vi "controlVoltagesCalc.vi"(0 "Camera":T1 {"InClusTiming 2"."TriggerMode" items=["Auto", "Software", "External sequence start ", "External exposure control"]; "InClusTiming 2"."ExposureTimeBase" items=["nanoseconds", "microseconds", "milliseconds"]; "InClusTiming 2"."Pixelclock" min=1 max=150 step=1 scale=0.05915..150.0; "InClusTiming 2"."Framerate" min=0.05915 max=2000.0 step=1.0 scale=0.05915..100.0 scale format="%#.3g"; "InClusTiming 2"."Exposure" min=0.001 max=400.0 step=0.001 scale=0.05915..400.0 scale format="%#.3g"}, 7 "clustPointagFin":T2, 11 "error in (no error)":errorcluster) -> (4 "output cluster":T1={"Camera.lvclass"=refnum, "InClusTiming 2"={"Pixelclock"=24, "Exposure"=46.39115, "ExposureTimeBase"=2, "Framerate"=14.99615, "TriggerMode"=0}, "ROI"={"PosX"=0, "PosY"=0, "Width"=0, "Height"=0}, "File Path Control"=path "", "mirror.lvclass"=refnum} {"InClusTiming 2"."TriggerMode" items=["Auto", "Software", "External sequence start ", "External exposure control"]; "InClusTiming 2"."ExposureTimeBase" items=["nanoseconds", "microseconds", "milliseconds"]; "InClusTiming 2"."Pixelclock" min=1 max=150 step=1 scale=0.05915..150.0; "InClusTiming 2"."Framerate" min=0.05915 max=2000.0 step=1.0 scale=0.05915..100.0 scale format="%#.3g"; "InClusTiming 2"."Exposure" min=0.001 max=400.0 step=0.001 scale=0.05915..400.0 scale format="%#.3g"}, 8 "clustPointagFin":T2, 15 "error out":errorcluster)   [LabVIEW 2020, in "Acquisition.lvlib"]
doc: "Perform the acquisition. Replace the contents of this diagram with calls to acquisition hardware."
uses:
  Acquisition.lvlib
  CLASS/Image Acquisition Class/Camera.lvclass
  MIRROR/mirror.lvclass
  SETTING/clustOA.ctl
  <vilib>/Analysis/Matrix/Datatypes/RealMatrix.ctl
  HardwareConfiguration.ctl
  <vilib>/Analysis/Matrix/Numeric/Conversions/Array To Matrix - RA.vi
  <vilib>/Analysis/Matrix/Numeric/Multiply/Multiply - RM,RM.vi
  <vilib>/Analysis/Matrix/Numeric/Conversions/Matrix To Array - RM.vi
  <vilib>/Analysis/Matrix/NI_Matrix.lvlib
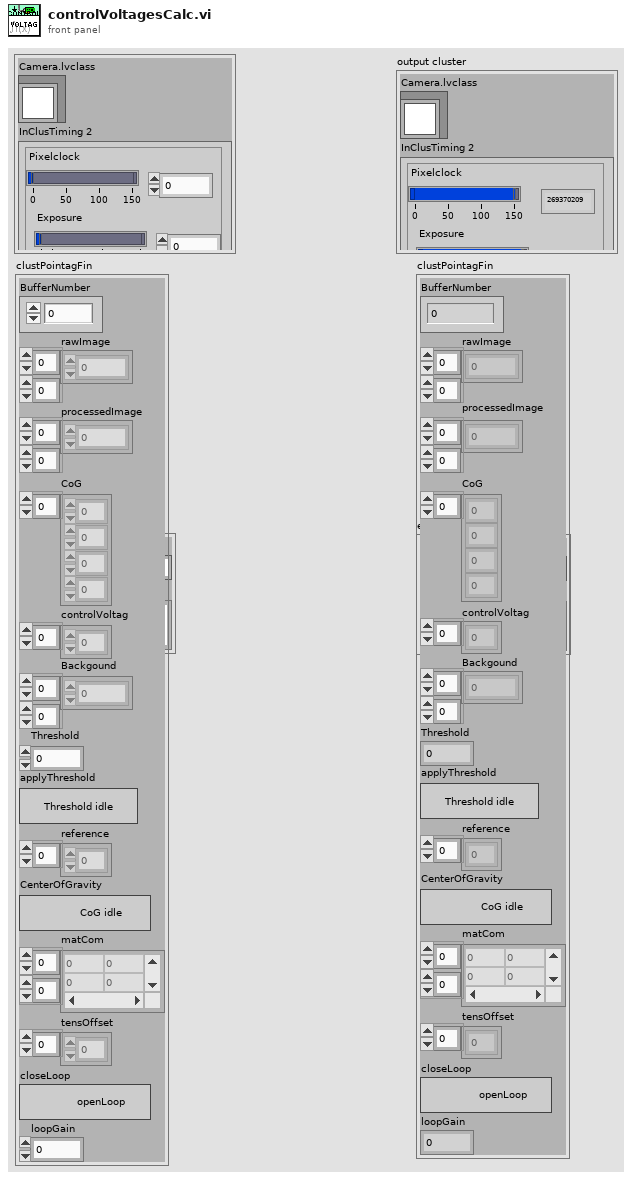
[diagram p1: front panel]
types:
  T1 = typedef "Acquisition.lvlib/HardwareConfiguration.ctl" = cluster{"Camera.lvclass":refnum<class "Camera.lvclass">, "InClusTiming 2":cluster{"Pixelclock":i32, "Exposure":dbl, "ExposureTimeBase":u16, "Framerate":dbl, "TriggerMode":u16}, "ROI":cluster{"PosX":i32, "PosY":i32, "Width":i32, "Height":i32}, "File Path Control":path, "mirror.lvclass":refnum<class "mirror.lvclass">}
  T2 = typedef "clustOA.ctl" = cluster{"BufferNumber":u32, "rawImage":u16[][], "processedImage":sgl[][], "CoG":dbl[], "controlVoltag":dbl[], "Backgound":sgl[][], "Threshold":dbl, "applyThreshold":bool, "reference":dbl[], "CenterOfGravity":bool, "matCom":T3, "tensOffset":dbl[], "closeLoop":bool, "loopGain":dbl}
  T3 = typedef "NI_Matrix.lvlib/RealMatrix.ctl" = dbl[][]
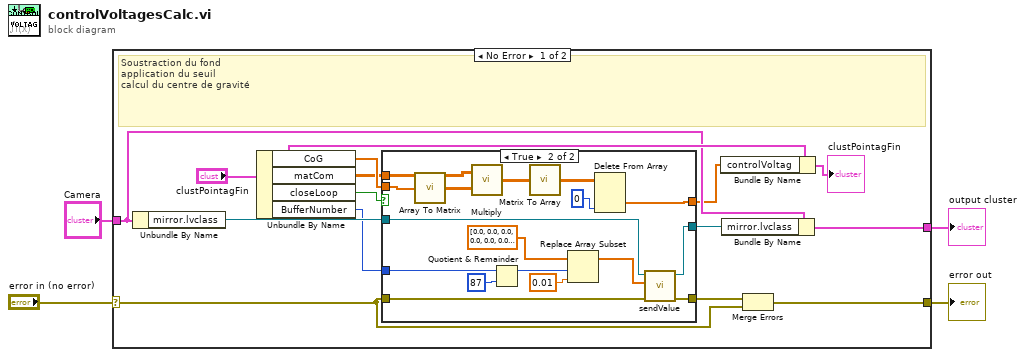
[diagram p0: block diagram]
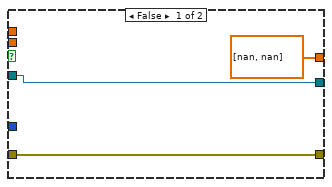
[diagram p2: hidden frame]
diagram:
  n1 = case shown="No Error" "error in (no error)" {
    selector: "error in (no error)" -> [w14 w40]
    tunnel: [w18 w40] -> w3
    tunnel: "Camera" -> [w10 w39]
    tunnel: [w9 w39] -> w1
    frame No Error {
      # "Soustraction du fond\napplication du seuil\ncalcul du centre de gravité"
      n2 = Unbundle By Name(w10) -> ("mirror.lvclass"=w8:refnum<class "mirror.lvclass">)
      n3 = Unbundle By Name("clustPointagFin") -> ("CoG"=w13:dbl[], "matCom"=w12:T3, "closeLoop"=w17:bool, "BufferNumber"=w5:u32)
      n4 = case shown="True" w17 {
        tunnel: w14 -> [w21 w38]
        tunnel: w13 -> [_ w32]
        tunnel: [w21 w25] -> w11
        tunnel: w12 -> [_ w33]
        tunnel: w8 -> [w20 w27]
        tunnel: [w20 w26] -> w7
        tunnel: [dbl[] [nan, nan] ("array") w23] -> w6
        tunnel: w5 -> [_ w22]
        frame False {
        }
        frame True {
          n5 = call-poly <vilib>:"Array To Matrix.vi"("Real 1D Array"=w32) -> ("Real Matrix (Column Vector)"=w37:T3)
          n6 = call-poly <vilib>:"Multiply.vi"("Real Matrix B"=w37, "Real Matrix A"=w33) -> ("A * B"=w36:T3)
          n7 = Quotient & Remainder(x=w22, y=87) -> (x-y*floor(x/y)=w31:u32)  [unwired: 1 out]
          n8 = call-poly <vilib>:"Matrix To Array.vi"("Real Matrix"=w36) -> ("Real 2D Array"=w35:dbl[][])
          n9 = Replace Array Subset(array=dbl[] [0.0, 0.0, 0.0, 0.0, 0.0, 0.0, 0.0, 0.0, 0.0, 0.0, 0.0, 0.0, 0.0, 0.0, 0.0, 0.0, 0.0, 0.0, 0.0, 0.0, 0.0, 0.0, 0.0, 0.0, 0.0, 0.0, 0.0, 0.0, 0.0, 0.0, 0.0, 0.0, 0.0, 0.0, 0.0, 0.0, 0.0, 0.0, 0.0, 0.0, 0.0, 0.0, 0.0, 0.0, 0.0, 0.0, 0.0, 0.0, 0.0, 0.0, 0.0, 0.0, 0.0, 0.0, 0.0, 0.0, 0.0, 0.0, 0.0, 0.0, 0.0, 0.0, 0.0, 0.0, 0.0, 0.0, 0.0, 0.0, 0.0, 0.0, 0.0, 0.0, 0.0, 0.0, 0.0, 0.0, 0.0, 0.0, 0.0, 0.0, 0.0, 0.0, 0.0, 0.0, 0.0, 0.0, 0.0, 0.0], new element=0.01 ("new element/subarray"), index=w31) -> (w24:dbl[])
          n10 = Delete From Array(array=w35, index (col)=0 ("index")) -> (deleted portion=w23:dbl[])  [unwired: 2 in, 1 out]
          n11 = call-dynamic "sendValue.vi"("error in (no error)"=w38, "value"=w24, "mirror in"=w27) -> ("error out"=w25:errorcluster, "mirror out"=w26:refnum<class "mirror.lvclass">)  [unwired: 7 in]
        }
      }
      n12 = Bundle By Name(cluster="clustPointagFin", "controlVoltag"=w6) -> (→"clustPointagFin":T2)
      n13 = Bundle By Name(cluster=w10, "mirror.lvclass"=w7) -> (w9:T1)
      n14 = Merge Errors(w11, w14) -> (w18:errorcluster)
    }
    frame Error {
    }
  }
  "error out" <- w3
  "output cluster" <- w1
